vi "Test_SHT21.vi"() -> ()   [LabVIEW 2014]
uses:
  <vilib>/MakerHub/LINX/Public/Utilities/Open Local.vi
  SHT21_class/SHT21.lvclass
  <vilib>/MakerHub/LINX/LMH-LINX.lvlib
panel:
  out "Data 2":u8[](array[numeric])
  out "RH":dbl
  out "Lynx Setup error":errorcluster
  out "Data":u8[](array[numeric])
  in  "stop":bool
  out "Temperature":dbl
  out "Error Out":errorcluster
  out "Device Name":string
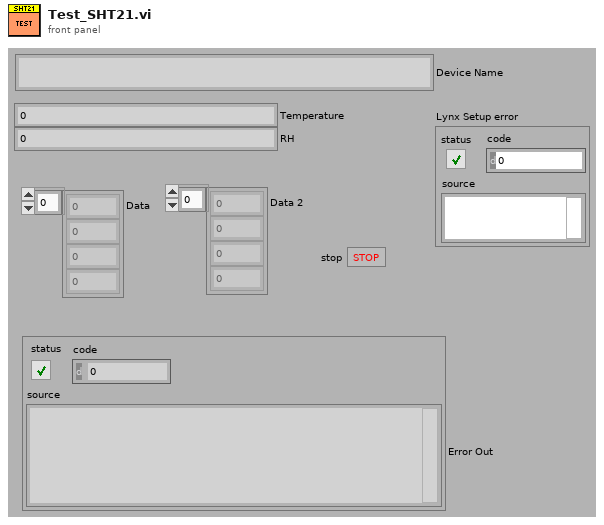
[diagram p1: front panel]
types:
  T1 = typedef "LMH-LINX.lvlib/LINX Ref.ctl" = cluster{"IO":T2, "Interface":T3, "LINX Device Config":T4}
  T2 = typedef "LMH-LINX.lvlib/Platform.ctl" = enum16{"Remote", "Local"}
  T3 = typedef "LMH-LINX.lvlib/Interface.ctl" = enum16{"Serial", "TCP"}
  T4 = typedef "LMH-LINX.lvlib/Device.lvlib/LINX Device Config.ctl" = cluster{"Interface":T3, "COM Port":refnum<visa-resource-name>, "TCP Configuration":T5, "Device Family":u8, "Device ID":u8, "Device Name":string, "TCP Ref":refnum<k5>, "Channels":T6}
  T5 = typedef "LMH-LINX.lvlib/Device.lvlib/TCP Config.ctl" = cluster{"IP Address":string, "Port":u16}
  T6 = typedef "LMH-LINX.lvlib/Channels.ctl" = cluster{"DI":u8[], "DO":u8[], "AI":u8[], "AO":u8[], "PWM":u8[], "QE":u8[], "UART":u8[], "I2C 2":u8[], "SPI":u8[], "CAN":u8[], "Servo":u8[], "AI Ref (V)":dbl, "AI Resolution (Bits)":u8, "AO Ref (V)":dbl, "AO Resolution (Bits)":u8}
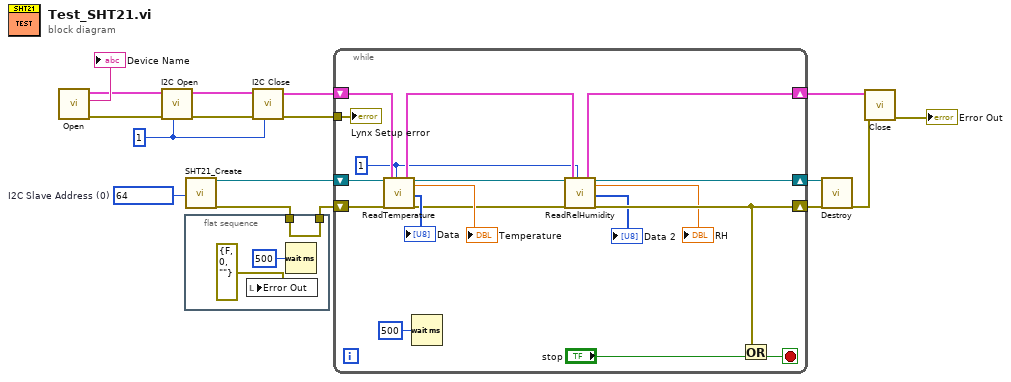
[diagram p0: block diagram]
diagram:
  w13 = u8 64  # I2C Slave Address (0)
  w5 = u8 1 ("I2C Channel (0)")
  n1 = call-poly <vilib>:"Open.vi"() -> ("Error Out"=w3:errorcluster, "Device Name"=→"Device Name":string, "LINX Resource"=w7:T1)  [unwired: 9 in]
  n2 = call <vilib>:"I2C Open.vi"("I2C Channel (0)"=w5, "Error In"=w3, "LINX Resource"=w7) -> ("Error Out"=w4:errorcluster, "LINX Resource"=w6:T1)  [unwired: 7 in]
  n3 = flat-sequence {
    tunnel: [w19] -> w12
    tunnel: w10 -> [w19]
    frame #0 {
      n4 = local write "Error Out"(errorcluster {"status"=FALSE, "code"=0, "source"=""} ("Error Out")) -> ()
      n5 = Wait (ms)(milliseconds to wait=u32 500) -> ()  [unwired: 1 out]
    }
  }
  n6 = call "SHT21_Create.vi"("I2C Slave Address (0)"=w13) -> ("reference out"=w9:refnum<class "SHT21.lvclass">, "error out"=w10:errorcluster)  [unwired: 17 in]
  n7 = call <vilib>:"I2C Close.vi"("I2C Channel (0)"=w5, "Error In"=w4, "LINX Resource"=w6) -> ("Error Out"=w2:errorcluster, "LINX Resource"=w8:T1)  [unwired: 7 in]
  n8 = while {
    shift-right: [w26] -> w17
    shift-left: w9 -> [w35]
    shift-right: [w27] -> w16
    shift-left: w12 -> [w34]
    shift-right: [w24] -> w11
    shift-left: w8 -> [w33]
    tunnel: w2 -> [w36]
    stop <- w37 stop-if-true
    w23 = u8 1 ("I2C Channel (0)")
    n9 = call-dynamic "ReadTemperature.vi"("reference in"=w35, "error in (no error)"=w34, "LINX Resource"=w33, "I2C Channel (0)"=w23) -> ("LINX Resource"=w25:T1, "reference out"=w29:refnum<class "SHT21.lvclass">, "Temperature"=→"Temperature":dbl, "Data Temp"=→"Data":u8[], "error out"=w28:errorcluster)  [unwired: 11 in]
    n10 = Wait (ms)(milliseconds to wait=u32 500) -> ()  [unwired: 1 out]
    n11 = call-dynamic "ReadRelHumidity.vi"("reference in"=w29, "error in (no error)"=w28, "LINX Resource"=w25, "I2C Channel (0)"=w23) -> ("LINX Resource"=w24:T1, "reference out"=w26:refnum<class "SHT21.lvclass">, "RH"=→"RH":dbl, "Data RH"=→"Data 2":u8[], "error out"=w27:errorcluster)  [unwired: 11 in]
    n12 = Or(x=w27, y="stop") -> (x .or. y?=w37:bool)
    "Lynx Setup error" <- w36
  }
  n13 = call-dynamic "Destroy.vi"("reference in"=w17, "error in (no error)"=w16) -> ("error out"=w1:errorcluster)  [unwired: 16 in, 1 out]
  n14 = call <vilib>:"Close.vi"("Error In"=w1, "LINX Resource"=w11) -> ("Error Out"=→"Error Out":errorcluster)  [unwired: 9 in]
